vi "ILC.vi"(4 "Force_mode_L":bool, 5 "L_NUM":u32, 6 "Force_mode_R":bool, 7 "R_NUM":u32, 8 "문자열":string="Auto_control", 9 "Target_Cur_L":i32, 10 "Targer_Cur_R":i32, 11 "ILC coefficient":sgl) -> (1 "Target_Cur_L":i32, 2 "Target_cur_R":i32)   [LabVIEW 2019]
uses:
  9b78af20-2324-4b2c-92e7-d14e661ccd4c.vi
  99d1b62b-bbe1-4d7a-89f1-36c93a09e13c.vi
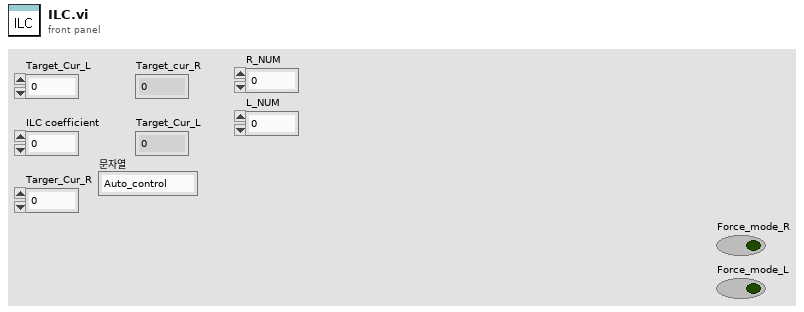
[diagram p1: front panel]
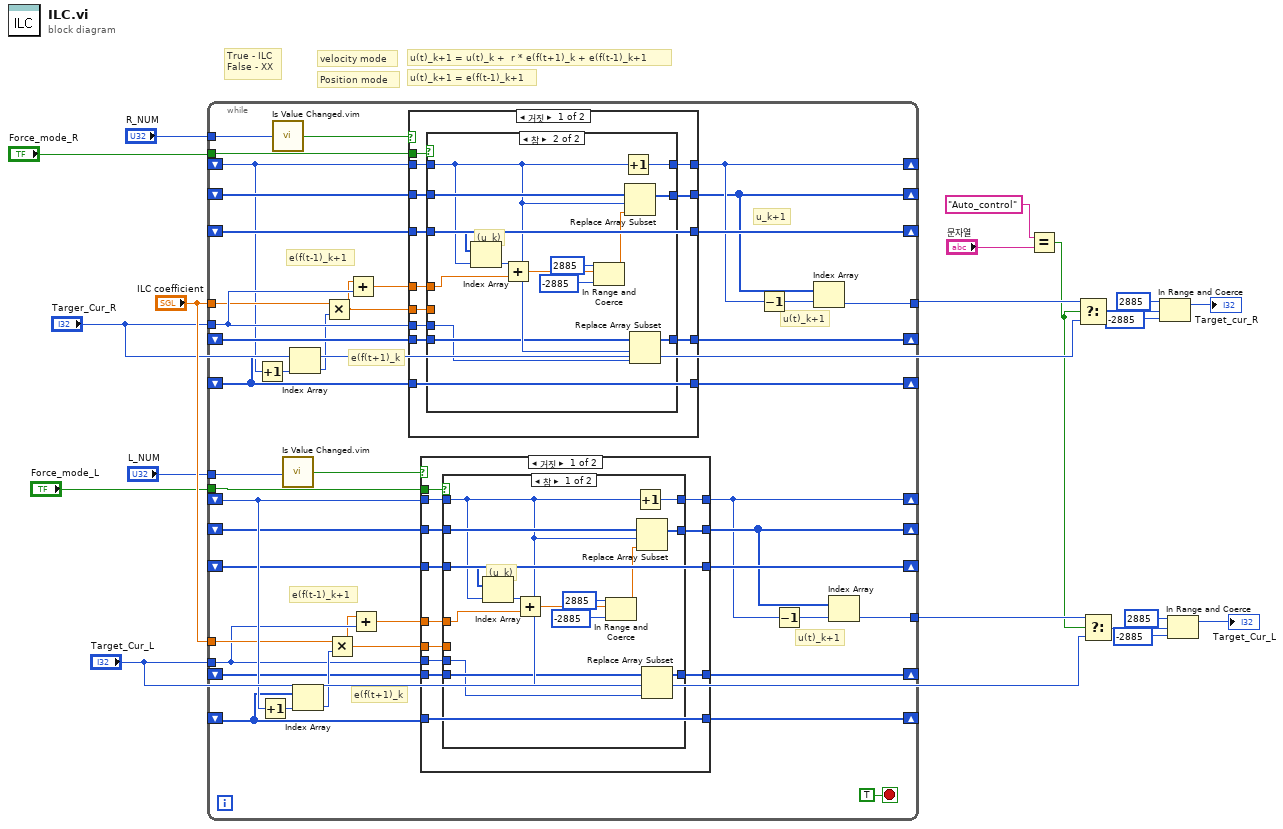
[diagram p0: block diagram]
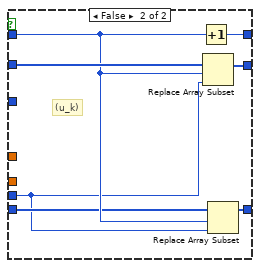
[diagram p2: hidden frame]
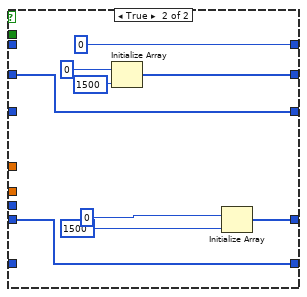
[diagram p3: hidden frame]
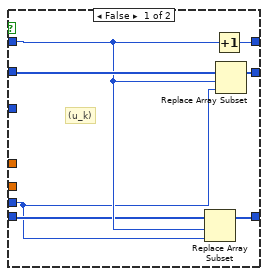
[diagram p4: hidden frame]
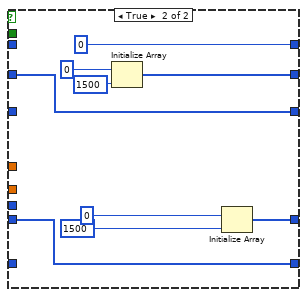
[diagram p5: hidden frame]
diagram:
  # "velocity mode"
  # "Position mode"
  # "u(t)_k+1 = e(f(t-1)_k+1"
  # "u(t)_k+1 = u(t)_k +  r * e(f(t+1)_k + e(f(t-1)_k+1"
  # "True - ILC\nFalse - XX"
  n1 = while {
    shift-right: [w59] -> _
    shift-left: _ -> [w46]
    shift-right: [w55] -> _
    shift-left: _ -> [w62]
    shift-right: [w60] -> _
    shift-left: _ -> [w61]
    tunnel: "Targer_Cur_R" -> [w51]
    tunnel: [w56] -> w15
    shift-right: [w54] -> _
    shift-left: _ -> [w53]
    shift-right: [w52] -> _
    shift-left: _ -> [w50]
    tunnel: "ILC coefficient" -> [w49]
    tunnel: "ILC coefficient" -> [w35]
    shift-right: [w43] -> _
    shift-left: _ -> [w37]
    tunnel: "Target_Cur_L" -> [w34]
    shift-right: [w30] -> _
    shift-left: _ -> [w42]
    shift-right: [w31] -> _
    shift-left: _ -> [w41]
    shift-right: [w40] -> _
    shift-left: _ -> [w39]
    shift-right: [w38] -> _
    shift-left: _ -> [w36]
    tunnel: [w29] -> w13
    tunnel: "L_NUM" -> [w26]
    tunnel: "R_NUM" -> [w25]
    tunnel: "Force_mode_R" -> [w24]
    tunnel: "Force_mode_L" -> [w23]
    stop <- TRUE stop-if-true
    # "u(t)_k+1"
    # "e(f(t-1)_k+1"
    # "e(f(t+1)_k"
    # "e(f(t-1)_k+1"
    # "u(t)_k+1"
    # "u_k+1"
    # "e(f(t+1)_k"
    n2 = Increment(x=w46) -> (x+1=w47:i32)
    n3 = Increment(x=w42) -> (x+1=w45:i32)
    n4 = call "Is Value Changed.vim"("value"=w25) -> ("changed or first call?"=w28:bool)
    n5 = call "Is Value Changed.vim"("value"=w26) -> ("changed or first call?"=w27:bool)
    n6 = Index Array(array=w50, index=w47) -> (element=w48:i32)
    n7 = Index Array(array=w36, index=w45) -> (element=w44:i32)
    n8 = Multiply(x=w49, y=w48) -> (x*y=w22:sgl)
    n9 = Multiply(x=w35, y=w44) -> (x*y=w21:sgl)
    n10 = Add(x=w22, y=w51) -> (x+y=w57:sgl)
    n11 = Add(x=w21, y=w34) -> (x+y=w33:sgl)
    n12 = case shown="거짓" w28 {
      tunnel: [w117 w145] -> w55
      tunnel: [w115 0 ("32비트 정수")] -> w59
      tunnel: w46 -> [w112 _]
      tunnel: w62 -> [w116 w144]
      tunnel: [w114 w144] -> w60
      tunnel: w61 -> [w114 _]
      tunnel: w57 -> [w113 _]
      tunnel: [w110 w140] -> w54
      tunnel: w53 -> [w111 w139]
      tunnel: [w108 w139] -> w52
      tunnel: w50 -> [w108 _]
      tunnel: w51 -> [w109 _]
      tunnel: w24 -> [w107 _]
      tunnel: w22 -> [w106 _]
      frame False {
        n13 = case shown="참" w107 {
          tunnel: [w121 w138] -> w117
          tunnel: w116 -> [w124 w137]
          tunnel: [w122 w136] -> w115
          tunnel: w114 -> [_ w135]
          tunnel: w113 -> [_ w125]
          tunnel: w112 -> [w123 w134]
          tunnel: w111 -> [w120 w133]
          tunnel: [w118 w132] -> w110
          tunnel: w109 -> [w119 w131]
          tunnel: w106 -> [_ _]
          frame False {
            # "(u_k)"
            n14 = Replace Array Subset(array=w120, new element=w119, index=w123) -> (w118:i32[])
            n15 = Increment(x=w123) -> (x+1=w122:i32)
            n16 = Replace Array Subset(array=w124, new element=w119, index=w123) -> (w121:i32[])
          }
          frame True {
            # "(u_k)"
            n17 = Index Array(array=w135, index=w134) -> (element=w130:i32)
            n18 = Add(x=w130, y=w125) -> (x+y=w127:sgl)
            n19 = In Range and Coerce(upper limit=2885 ("상위 리미트"), x=w127, lower limit=-2885 ("하위 리미트")) -> (coerced(x)=w126:sgl)  [unwired: 1 out]
            n20 = Increment(x=w134) -> (x+1=w136:i32)
            n21 = Replace Array Subset(array=w137, new element=w126, index=w134) -> (w138:i32[])
            n22 = Replace Array Subset(array=w133, new element=w131, index=w134) -> (w132:i32[])
          }
        }
      }
      frame True {
        n23 = Initialize Array(0 ("32비트 정수"), 1500 ("차원 크기")) -> (w145:i32[])
        n24 = Initialize Array(0 ("32비트 정수"), 1500 ("차원 크기")) -> (w140:i32[])
      }
    }
    n25 = case shown="거짓" w27 {
      tunnel: [w75 w103] -> w31
      tunnel: [w73 0 ("32비트 정수")] -> w30
      tunnel: w42 -> [w71 _]
      tunnel: w41 -> [w74 w102]
      tunnel: [w72 w102] -> w40
      tunnel: w39 -> [w72 _]
      tunnel: w33 -> [w66 _]
      tunnel: [w69 w98] -> w43
      tunnel: w37 -> [w70 w97]
      tunnel: [w67 w97] -> w38
      tunnel: w36 -> [w67 _]
      tunnel: w34 -> [w68 _]
      tunnel: w23 -> [w65 _]
      tunnel: w21 -> [w64 _]
      frame False {
        n26 = case shown="참" w65 {
          tunnel: [w89 w96] -> w75
          tunnel: w74 -> [w88 w95]
          tunnel: [w87 w94] -> w73
          tunnel: w72 -> [w86 _]
          tunnel: w71 -> [w85 w93]
          tunnel: w70 -> [w84 w92]
          tunnel: [w83 w91] -> w69
          tunnel: w68 -> [w82 w90]
          tunnel: w66 -> [w76 _]
          tunnel: w64 -> [_ _]
          frame True {
            # "(u_k)"
            n27 = Index Array(array=w86, index=w85) -> (element=w81:i32)
            n28 = Add(x=w81, y=w76) -> (x+y=w78:sgl)
            n29 = In Range and Coerce(upper limit=2885 ("상위 리미트"), x=w78, lower limit=-2885 ("하위 리미트")) -> (coerced(x)=w77:sgl)  [unwired: 1 out]
            n30 = Increment(x=w85) -> (x+1=w87:i32)
            n31 = Replace Array Subset(array=w88, new element=w77, index=w85) -> (w89:i32[])
            n32 = Replace Array Subset(array=w84, new element=w82, index=w85) -> (w83:i32[])
          }
          frame False {
            # "(u_k)"
            n33 = Increment(x=w93) -> (x+1=w94:i32)
            n34 = Replace Array Subset(array=w95, new element=w90, index=w93) -> (w96:i32[])
            n35 = Replace Array Subset(array=w92, new element=w90, index=w93) -> (w91:i32[])
          }
        }
      }
      frame True {
        n36 = Initialize Array(0 ("32비트 정수"), 1500 ("차원 크기")) -> (w103:i32[])
        n37 = Initialize Array(0 ("32비트 정수"), 1500 ("차원 크기")) -> (w98:i32[])
      }
    }
    n38 = Decrement(x=w59) -> (x-1=w58:i32)
    n39 = Decrement(x=w30) -> (x-1=w32:i32)
    n40 = Index Array(array=w55, index=w58) -> (element=w56:i32)
    n41 = Index Array(array=w31, index=w32) -> (element=w29:i32)
  }
  n42 = Equal?(x="Auto_control", y="문자열") -> (x = y?=w11:bool)
  n43 = Select(t=w15, s=w11, f="Targer_Cur_R") -> (s? t:f=w8:i32)
  n44 = Select(t=w13, s=w11, f="Target_Cur_L") -> (s? t:f=w4:i32)
  n45 = In Range and Coerce(upper limit=2885 ("상위 리미트"), x=w8, lower limit=-2885 ("하위 리미트")) -> (coerced(x)=→"Target_cur_R":i32)  [unwired: 1 out]
  n46 = In Range and Coerce(upper limit=2885 ("상위 리미트"), x=w4, lower limit=-2885 ("하위 리미트")) -> (coerced(x)=→"Target_Cur_L":i32)  [unwired: 1 out]
